vi "Initailize.vi"(8 "error in (no error)":errorcluster, 9 "zeromq.lvlib:ZeroMQ Context":refnum<class "zmq_context.lvclass">, 10 "Name":string, 11 "Channel Rep in":refnum<class "Channel Rep.lvclass">) -> (0 "error out":errorcluster, 3 "Channel Rep out":refnum<class "Channel Rep.lvclass">)   [LabVIEW 2018, in "Channel Rep.lvclass"]
uses:
  Channel Rep.lvclass
  <vilib>/addons/zeromq/zmq_context.lvclass
  Communication Channel/Communication Channel.lvclass
  Socket/Socket.lvclass
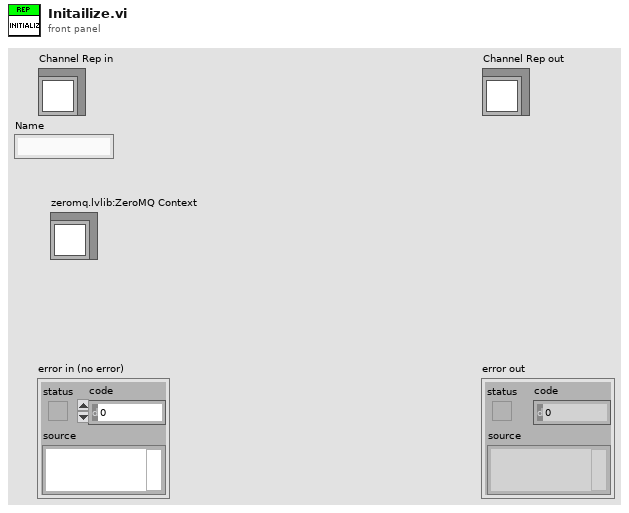
[diagram p1: front panel]
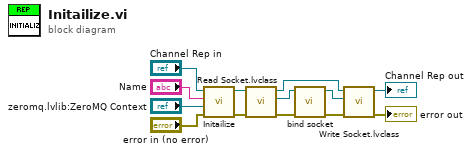
[diagram p0: block diagram]
diagram:
  n1 = call-parent "Initailize.vi"("error in (no error)"="error in (no error)", "zeromq.lvlib:ZeroMQ Context"="zeromq.lvlib:ZeroMQ Context", "Name"="Name", "Communication Channel in"="Channel Rep in") -> ("error out"=w8:errorcluster, "Communication Channel out"=w9:refnum<class "Channel Rep.lvclass">)  [unwired: 6 in]
  n2 = call-dynamic "Read Socket.lvclass.vi"("error in (no error)"=w8, "Communication Channel in"=w9) -> ("error out"=w1:errorcluster, "Socket.lvclass"=w4:refnum<class "Socket.lvclass">, "Communication Channel out"=w7:refnum<class "Channel Rep.lvclass">)  [unwired: 7 in]
  n3 = call "bind socket.vi"("error in (no error)"=w1, "Socket in"=w4) -> ("error out"=w2:errorcluster, "Socket out"=w3:refnum<class "Socket.lvclass">)  [unwired: 8 in]
  n4 = call-dynamic "Write Socket.lvclass.vi"("error in (no error)"=w2, "Socket2.lvclass"=w3, "Communication Channel in"=w7) -> ("error out"=→"error out":errorcluster, "Communication Channel out"=→"Channel Rep out":refnum<class "Channel Rep.lvclass">)  [unwired: 7 in]
